vi "EnqueSequence(CommandOnly).vi"(7 "at front (F)":bool, 8 "error in":errorcluster, 10 "Message Commands":string[](array[string]), 11 "Message que":T1) -> (0 "error out":errorcluster, 3 "Message que out":T1)   [LabVIEW 2019]
doc: "Transmit a message with a no payload.\nFor a regular message, enqueue the message. For a priority message, enqueue it at the front of the queue.\n\nBolder Software LLC"
uses:
  MessageQue/MessageQue.ctl
  MessageQue/MessageCluster.ctl
  MessageQue/MessageQue.lvlib
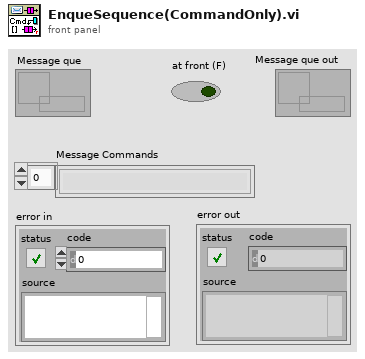
[diagram p1: front panel]
types:
  T1 = typedef "MessageQue.lvlib/MessageQue.ctl" = refnum<queue>
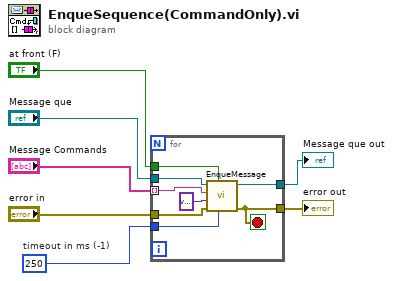
[diagram p0: block diagram]
diagram:
  w7 = 250  # timeout in ms (-1)
  n1 = for {
    tunnel: w7 -> [w15]
    tunnel: "at front (F)" -> [w14]
    tunnel: "Message Commands" -> [w11] mode=indexing
    tunnel: "Message que" -> [w13]
    tunnel: [w12] -> w4
    tunnel: "error in" -> [w10]
    tunnel: [w8] -> w1
    stop <- w8 stop-if-true
    n2 = call "EnqueMessage.vi"("timeout in ms (-1)"=w15, "Priority Message? (F)"=w14, "error in"=w10, "Message Payload"=variant, "Message Command"=w11, "Message que"=w13) -> ("error out"=w8:errorcluster, "Message que out"=w12:T1)  [unwired: 4 in]
  }
  "Message que out" <- w4
  "error out" <- w1
